vi "SimpleSphere.vi"(0 "Radius":sgl=0.05, 1 "Name":string, 2 "origin":T1, 3 "mass":dbl=1.0, 4 "link color":u32(colorbox)=16712704) -> (5 "Link":T2)   [LabVIEW 2012]
uses:
  <userlib>/rosforlv/Gazebo/URDF_conversion/LINK.ctl
  <userlib>/rosforlv/Gazebo/URDF_conversion/Position.ctl
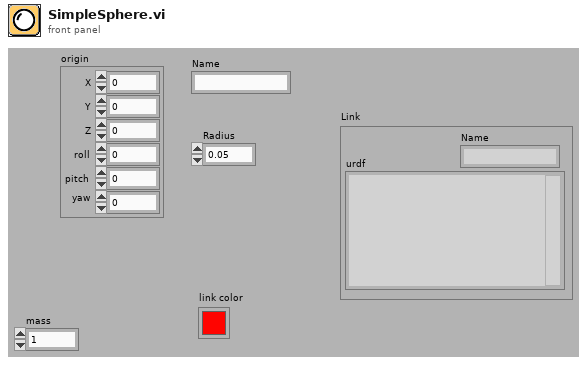
[diagram p1: front panel]
types:
  T1 = typedef "Position.ctl" = cluster{"X":sgl, "Y":sgl, "Z":sgl, "roll":sgl, "pitch":sgl, "yaw":sgl}
  T2 = typedef "LINK.ctl" = cluster{"Name":string, "urdf":string}
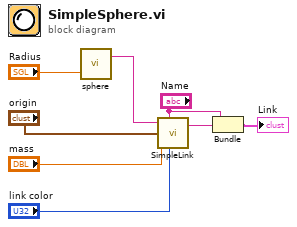
[diagram p0: block diagram]
diagram:
  n1 = call <userlib>:"sphere.vi"("Radius"="Radius") -> ("urdf out"=w7:string)  [unwired: 3 in]
  n2 = call <userlib>:"SimpleLink.vi"("Geometry"=w7, "Name"="Name", "origin"="origin", "mass"="mass", "link color"="link color") -> ("link out"=w3:string)  [unwired: 1 in]
  n3 = Bundle("Name"="Name", "link out"=w3) -> (→"Link":cluster{"Name":string, "link out":string})  [unwired: 1 in]
